vi "read_4ch.vi"(10 "channel offsets":T1) -> (2 "read output":T1)   [LabVIEW 2011]
uses:
  typedefs/channels_array.ctl
  typedefs/channel_decoding_enum.ctl
  <vilib>/rvi/eio/common/nirviEmuTemplateMethod_errors.vi
  <vilib>/eio/EIONode/EIONode.xnode
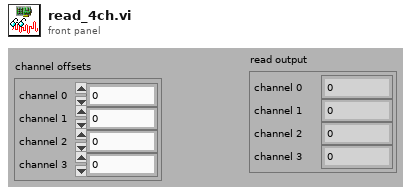
[diagram p1: front panel]
types:
  T1 = typedef "channels_array.ctl" = cluster{"channel 0":u32, "channel 1":u32, "channel 2":u32, "channel 3":u32}
  T2 = typedef "channel_decoding_enum.ctl" = enum16{"A", "B"}
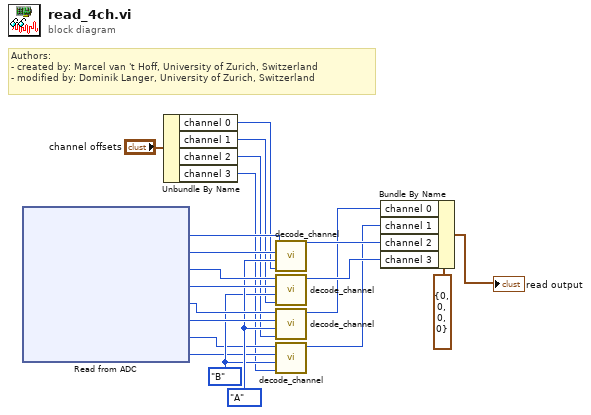
[diagram p0: block diagram]
diagram:
  w12 = channel_decoding_enum."B" ("channel decoding")
  w13 = channel_decoding_enum."A" ("channel decoding")
  # "Authors: \n- created by: Marcel van 't Hoff, University of Zurich, Switzerland\n- modified by: Dominik Langer, University of Zurich, Switzerland"
  n1 = xnode "Read from ADC"() -> ("Connector1/DIOPORT3"=w20:u8, "Connector1/DIOPORT2"=w19:u8, "Connector1/DIOPORT1"=w17:u8, "Connector1/DIOPORT0"=w16:u8, "Connector0/DIOPORT3"=w15:u8, "Connector0/DIOPORT2"=w14:u8, "Connector0/DIOPORT1"=w11:u8, "Connector0/DIOPORT0"=w10:u8)  [unwired: 8 in, 8 out]
  n2 = Unbundle By Name("channel offsets") -> ("channel 0"=w6:u32, "channel 1"=w5:u32, "channel 2"=w4:u32, "channel 3"=w3:u32)
  n3 = call "decode_channel.vi"("offset"=w6, "channel decoding"=w13, "port B"=w19, "port A"=w20) -> ("channel value"=w18:u32)  [unwired: 7 in]
  n4 = call "decode_channel.vi"("offset"=w5, "channel decoding"=w12, "port B"=w16, "port A"=w17) -> ("channel value"=w9:u32)  [unwired: 7 in]
  n5 = call "decode_channel.vi"("offset"=w4, "channel decoding"=w13, "port B"=w14, "port A"=w15) -> ("channel value"=w8:u32)  [unwired: 7 in]
  n6 = call "decode_channel.vi"("offset"=w3, "channel decoding"=w12, "port B"=w10, "port A"=w11) -> ("channel value"=w7:u32)  [unwired: 7 in]
  n7 = Bundle By Name(cluster=T1 {"channel 0"=0, "channel 1"=0, "channel 2"=0, "channel 3"=0} ("channel offsets 3"), "channel 0"=w8, "channel 1"=w7, "channel 2"=w18, "channel 3"=w9) -> (→"read output":T1)
